vi "Trigger.vi"(8 "error in (no error)":errorcluster, 10 "Command (0:Rem Trig)":T1(ring), 11 "VISA Resource Name":refnum<visa-resource-name>) -> (0 "error out":errorcluster, 3 "VISA Resource Name Out":refnum<visa-resource-name>)   [LabVIEW 2012, in "Agilent 34970.lvlib"]
doc: "This VI lets you trigger the instrument remotely (from your computer), place the instrument in \"wait for trigger\" state, or abort the scan."
uses:
  <instrlib>/Agilent 34970/Agilent 34970.lvlib
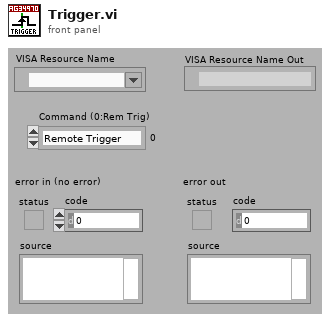
[diagram p1: front panel]
types:
  T1 = enum16{"Remote Trigger", "Immediate Trigger", "Wait for Trigger", "Abort Scan"}
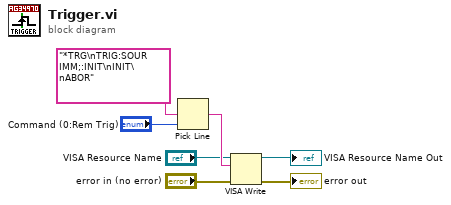
[diagram p0: block diagram]
diagram:
  n1 = Pick Line(multi-line string="*TRG\nTRIG:SOUR IMM;:INIT\nINIT\nABOR", line index="Command (0:Rem Trig)") -> (output string=w6:string)  [unwired: 1 in]
  n2 = VISA Write(VISA resource name="VISA Resource Name", write buffer=w6, error in (no error)="error in (no error)") -> (VISA resource name out=→"VISA Resource Name Out":refnum<visa-resource-name>, error out=→"error out":errorcluster)  [unwired: 1 out]
